vi "Heat_Load_Control.vi"(7 "Heat Load Control":enum32{"Catalyst 1 ", "Catalyst 2 ", "All"}(ring), 10 "Catalyst 2":dbl[](array[numeric]), 11 "Catalyst 1":dbl[](array[numeric])) -> (1 "Ki() Array":dbl[](array[numeric]), 2 "Control Cat":dbl)   [LabVIEW 2014]
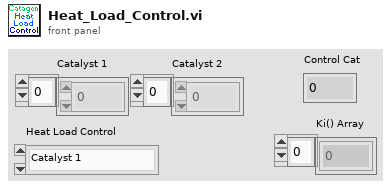
[diagram p1: front panel]
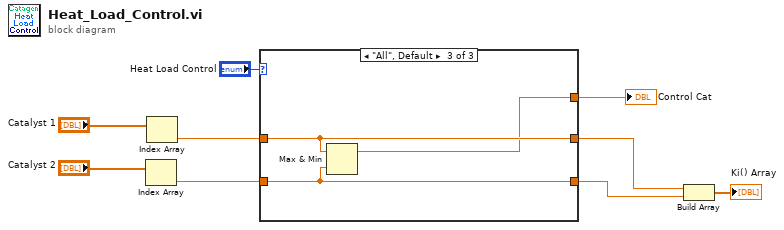
[diagram p0: block diagram]
diagram:
  n1 = Index Array(array="Catalyst 2") -> (element=w8:dbl)  [unwired: 1 in]
  n2 = Index Array(array="Catalyst 1") -> (element=w9:dbl)  [unwired: 1 in]
  n3 = case shown="\"All\", Default" "Heat Load Control" {
    tunnel: w9 -> [w10 w13 w16]
    tunnel: w8 -> [w11 w12 w15]
    tunnel: [w10 w13 w16] -> w4
    tunnel: [w11 w12 w15] -> w3
    tunnel: [w10 w12 w14] -> w5
    frame "Catalyst 1 " {
    }
    frame "Catalyst 2 " {
    }
    frame "All", Default {
      n4 = Max & Min(x=w16, y=w15) -> (max(x,y)=w14:dbl)  [unwired: 1 out]
    }
  }
  "Control Cat" <- w5
  n5 = Build Array(w4, w3) -> (→"Ki() Array":dbl[])
